vi "daqio_Put_Device_Type.vi"(8 "error in (no error)":errorcluster, 10 "device type in":T1, 11 "daq.io type in":T6={"daq.io ref"=refnum, "daq.io API Base"="http://dashboard.daq.io/api/v1", "Device Type Key"="", "Device Key"="", "Account ID"="", "online"=TRUE, "SSL"=TRUE}) -> (0 "error out":errorcluster, 3 "daq.io type out":T6={"daq.io ref"=refnum, "daq.io API Base"="http://dashboard.daq.io/api/v1", "Device Type Key"="", "Device Key"="", "Account ID"="", "online"=TRUE, "SSL"=TRUE})   [LabVIEW 2013, in "daqio minimal.lvlib"]
doc: "This VI updates a selected Device Type on this account according to the data on the input. Use this VI to update general changes to the device type. When adding new channels, events or tags, consider using the \"check and autocreate\" functions."
uses:
  daqio minimal.lvlib
  _typedefs/daqio-Type.ctl
  <vilib>/httpClient/ClientHandle.ctl
  _typedefs/daqio-Device-Type-Info-return.ctl
  _typedefs/daqio-Channel-Type-POST-return.ctl
  _typedefs/daqio-Device.ctl
  _typedefs/daqio-Event-Type.ctl
  _typedefs/daqio-Tag-Type-POST-return.ctl
  <vilib>/Easy HTTP Client/Easy HTTP.lvlib
  <vilib>/httpClient/LabVIEWHTTPClient.lvlib
panel:
  out "body":string
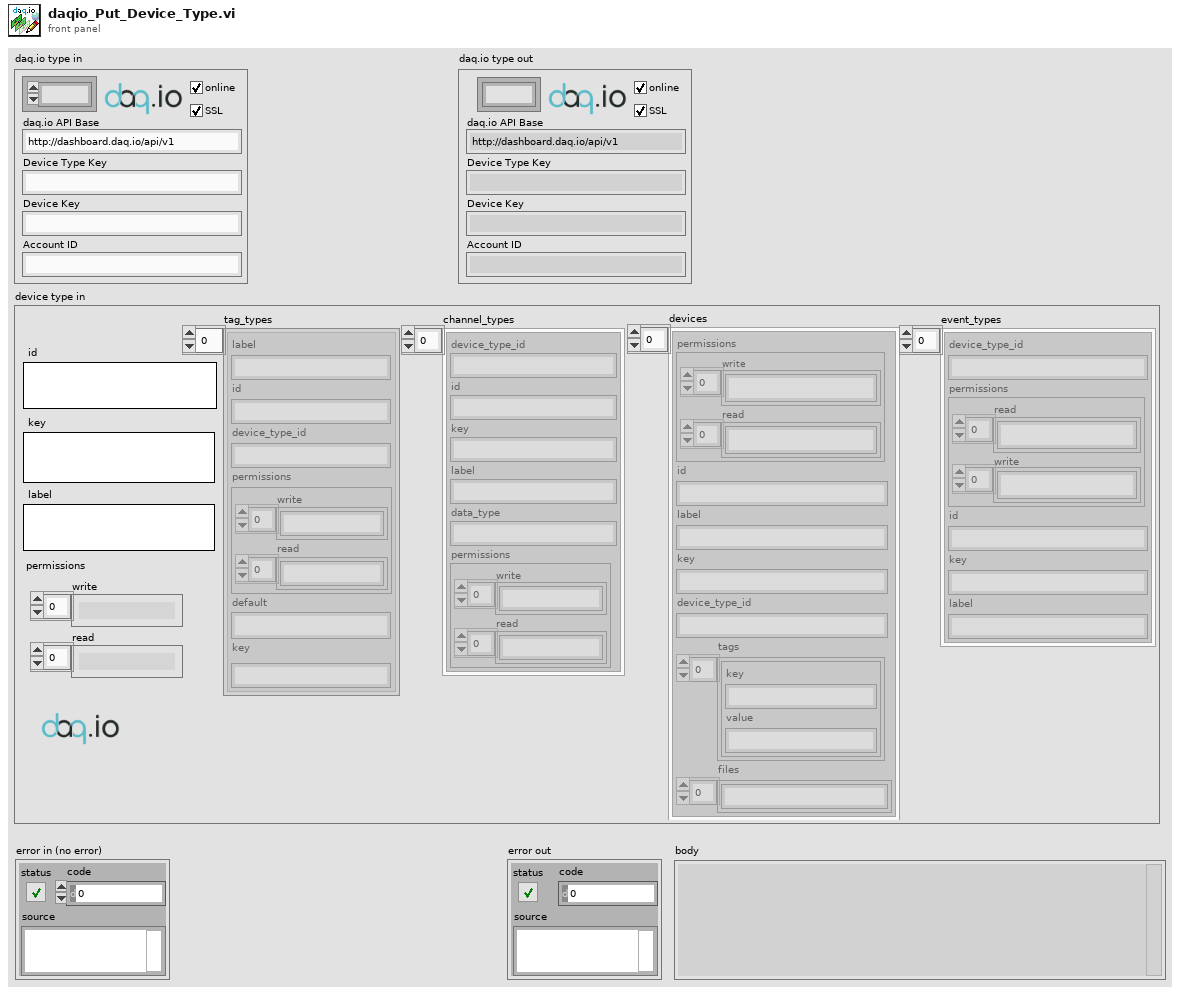
[diagram p1: front panel]
types:
  T1 = typedef "daqio minimal.lvlib/daqio-Device-Type-Info-return.ctl" = cluster{"channel_types":T2[], "devices":T3[], "label":string, "event_types":T4[], "key":string, "tag_types":T5[], "id":string, "permissions":cluster{"write":string[], "read":string[]}}
  T2 = typedef "daqio minimal.lvlib/daqio-Channel-Type-POST-return.ctl" = cluster{"device_type_id":string, "id":string, "key":string, "label":string, "data_type":string, "permissions":cluster{"write":string[], "read":string[]}}
  T3 = typedef "daqio minimal.lvlib/daqio-Device.ctl" = cluster{"permissions":cluster{"write":string[], "read":string[]}, "id":string, "label":string, "key":string, "device_type_id":string, "tags":cluster{"key":string, "value":string}[], "files":string[]}
  T4 = typedef "daqio minimal.lvlib/daqio-Event-Type.ctl" = cluster{"device_type_id":string, "permissions":cluster{"read":string[], "write":string[]}, "id":string, "key":string, "label":string}
  T5 = typedef "daqio minimal.lvlib/daqio-Tag-Type-POST-return.ctl" = cluster{"label":string, "id":string, "device_type_id":string, "permissions":cluster{"write":string[], "read":string[]}, "default":string, "key":string}
  T6 = typedef "daqio minimal.lvlib/daqio-Type.ctl" = cluster{"daq.io ref":T7, "daq.io API Base":string, "Device Type Key":string, "Device Key":string, "Account ID":string, "online":bool, "SSL":bool}
  T7 = typedef "LabVIEWHTTPClient.lvlib/ClientHandle.ctl" = refnum<k1>
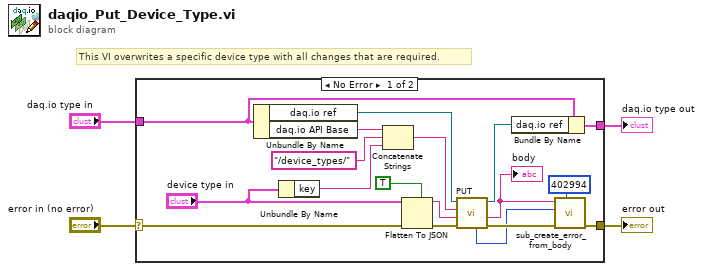
[diagram p0: block diagram]
diagram:
  # "This VI overwrites a specific device type with all changes that are required."
  n1 = case shown="No Error" "error in (no error)" {
    selector: "error in (no error)" -> [w14 w23]
    tunnel: "daq.io type in" -> [w22 w24]
    tunnel: [w21 w24] -> w3
    tunnel: [w9 w23] -> w2
    frame No Error {
      n2 = Unbundle By Name(w22) -> ("daq.io ref"=w20:T7, "daq.io API Base"=w18:string)
      n3 = Unbundle By Name("device type in") -> ("key"=w10:string)
      n4 = Concatenate Strings(w18, "/device_types/", w10) -> (w16:string)
      n5 = Flatten To JSON(enable LabVIEW extensions? (T)=TRUE, anything="device type in", error in (no error)=w14) -> (JSON string=w12:string, 11:w13:errorcluster)
      n6 = call <vilib>:"PUT.vi"("error in (no error)"=w13, "data"=w12, "url"=w16, "client handle"=w20) -> ("error out"=w8:errorcluster, "body"=w6:string, "client handle out"=w19:T7, "HTTP Response Code"=w7:i32)  [unwired: 3 in, 1 out]
      "body" <- w6
      n7 = Bundle By Name(cluster=w22, "daq.io ref"=w19) -> (w21:T6)
      n8 = call "sub_create_error_from_body.vi"("error code"=402994, "error in (no error)"=w8, "http code"=w7, "body"=w6) -> ("error out"=w9:errorcluster)  [unwired: 7 in]
    }
    frame Error {
    }
  }
  "error out" <- w2
  "daq.io type out" <- w3
